vi "timming_array_to_digital_waveform.vi"(2 "time unit":enum16{"s", "ms", "us", "ns"}(ring), 3 "delay array":dbl[](array[numeric]) format="%#_6e", 4 "resolution":i32=100) -> (0 "digital waveform":digitalwaveform(waveform)={"t0"=timestamp(0 s since 1904-01-01), "dt"=0.0, "Y"={"transitions"=[], "data"=[]}, "error"={"status"=FALSE, "code"=37421928, "source"=""}})   [LabVIEW 2011]
doc: "takes the timing info recieved from the DG645 Delay generator and transforms it into a digital waveform graph.\nMakes sure, all timings are setup in reference to t0!"
uses:
  <vilib>/Waveform/DWDTOps.llb/DWDT Boolean Array to Digital.vi
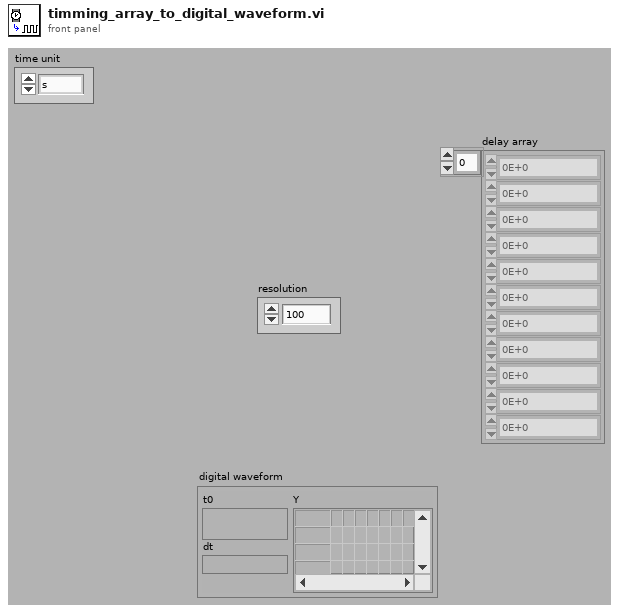
[diagram p1: front panel]
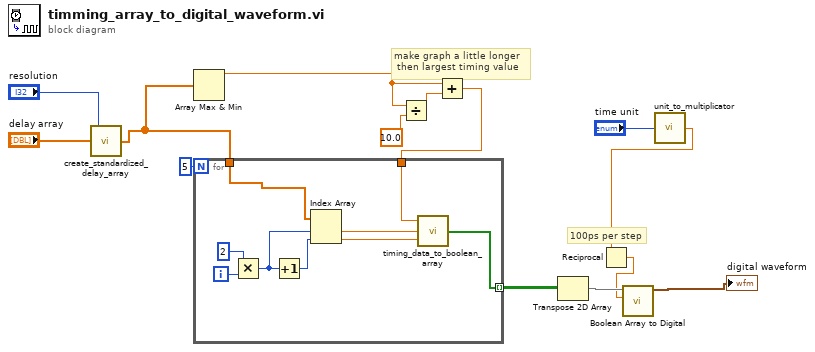
[diagram p0: block diagram]
diagram:
  # "100ps per step"
  # "make graph a little longer\n then largest timing value"
  n1 = call "create_standardized_delay_array.vi"("delay array"="delay array", "resolution"="resolution") -> ("standardize array"=w4:dbl[])  [unwired: 2 in, 1 out]
  n2 = Array Max & Min(array=w4) -> (max value=w7:dbl)  [unwired: 3 out]
  n3 = Divide(x=w7, y=10.0) -> (x/y=w10:dbl)
  n4 = Add(x=w7, y=w10) -> (x+y=w8:dbl)
  n5 = for {
    N: 5 -> [_]
    tunnel: [w21] -> w13 mode=indexing
    tunnel: w8 -> [w20]
    tunnel: w4 -> [w15]
    i -> [w23]
    n6 = Multiply(x=2, y=w23) -> (x*y=w16:i32)
    n7 = Increment(x=w16) -> (x+1=w19:i32)
    n8 = Index Array(array=w15, index #1=w16, index #2=w19) -> (element #1=w18:dbl, element #2=w17:dbl)
    n9 = call "timing_data_to_boolean_array.vi"("end time [us]"=w17, "start time [us]"=w18, "overall length [us]"=w20) -> ("boolean timing array"=w21:bool[])  [unwired: 1 in]
  }
  n10 = Transpose 2D Array(2D array=w13) -> (transposed array=w12:bool[][])
  n11 = call "unit_to_multiplicator.vi"("time unit"="time unit") -> ("multiplicator"=w1:dbl)
  n12 = Reciprocal(x=w1) -> (1/x=w9:dbl)
  n13 = call-poly <vilib>:"Boolean Array to Digital.vi"("sample rate"=w9, "boolean array"=w12) -> ("digital waveform"=→"digital waveform":digitalwaveform)  [unwired: 8 in, 1 out]
